vi "Write LINX I2C.vi"(8 "error in (no error)":errorcluster, 10 "LINX I2C":refnum<class "LINX I2C.lvclass">, 11 "TCS3472 in":refnum<class "TCS3472.lvclass">) -> (0 "error out":errorcluster, 3 "TCS3472 out":refnum<class "TCS3472.lvclass">)   [LabVIEW 2020, in "TCS3472.lvclass"]
uses:
  TCS3472.lvclass
  LINX I2C/LINX I2C.lvclass
  TCS3472.lvclass/TCS3472.ctl
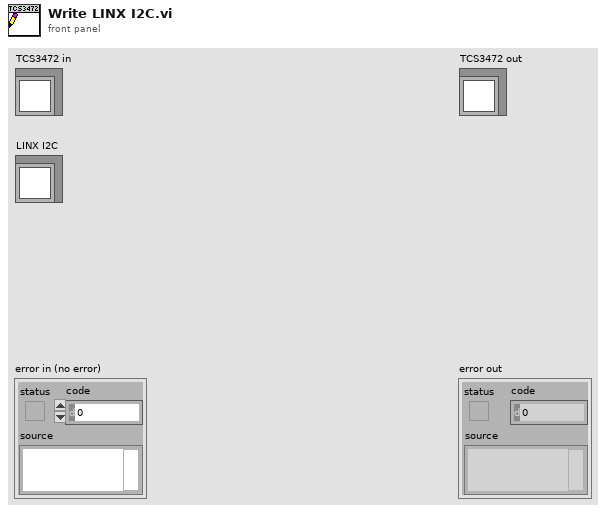
[diagram p1: front panel]
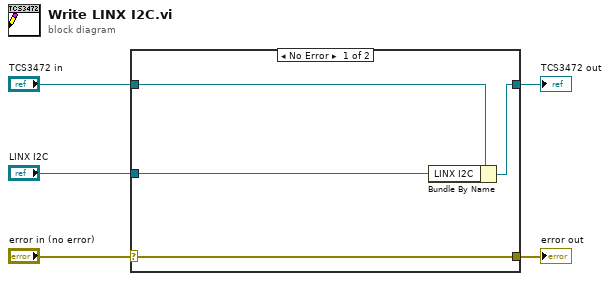
[diagram p0: block diagram]
diagram:
  n1 = case shown="No Error" "error in (no error)" {
    selector: "error in (no error)" -> [w9 w10]
    tunnel: [w9 w10] -> w4
    tunnel: [w7 w11] -> w2
    tunnel: "TCS3472 in" -> [w8 w11]
    tunnel: "LINX I2C" -> [w6 _]
    frame No Error {
      n2 = Bundle By Name(cluster=w8, "LINX I2C"=w6) -> (w7:refnum<class "TCS3472.lvclass">)
    }
    frame Error {
    }
  }
  "error out" <- w4
  "TCS3472 out" <- w2
